vi "StopServer.vi"(8 "error in (no error)":errorcluster, 11 "Server in":refnum<class "Server.lvclass">) -> (0 "error out":errorcluster, 2 "RunTime":u64, 3 "Server out":refnum<class "Server.lvclass">)   [LabVIEW 2017, in "opcua.lvlib" / "Server.lvclass"]
uses:
  Server.lvclass
  Server.lvclass/Server.ctl
  opcua32.dll
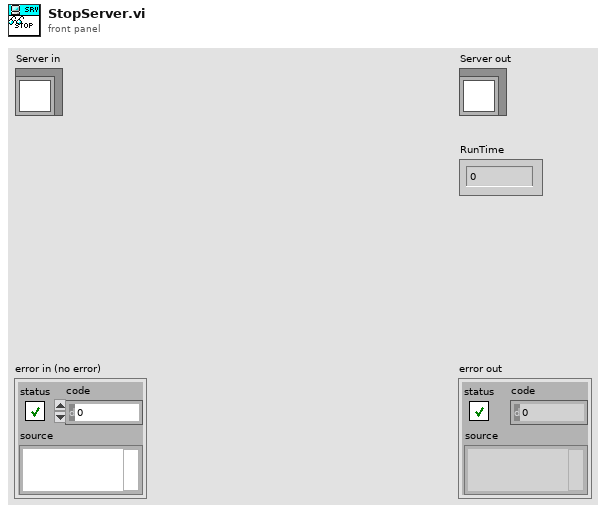
[diagram p1: front panel]
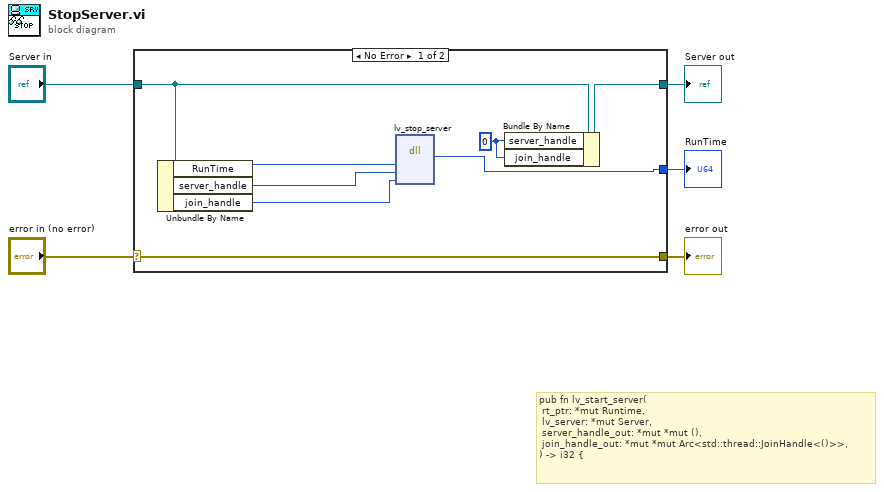
[diagram p0: block diagram]
diagram:
  # "pub fn lv_start_server(\n\trt_ptr: *mut Runtime,\n\tlv_server: *mut Server,\n\tserver_handle_out: *mut *mut (),\n\tjoin_handle_out: *mut *mut Arc<std::thread::JoinHandle<()>>,\n) -> i32 {"
  n1 = case shown="No Error" "error in (no error)" {
    selector: "error in (no error)" -> [w13 w14]
    tunnel: [w13 w14] -> w4
    tunnel: [w9 w15] -> w2
    tunnel: "Server in" -> [w10 w15]
    tunnel: [w8 _] -> w1
    frame No Error {
      w6 = u64 0 ("server_handle")
      n2 = Unbundle By Name(w10) -> ("RunTime"=w12:u64, "server_handle"=w11:u64, "join_handle"=w7:u64)
      n3 = dll-call lib="C:/Users/Andrey/Desktop/opcua-labview/opcua-lvlib/opcua*.dll" fn="lv_stop_server"("RunTime"=w12, "handle"=w11, "joi_handle"=w7) -> ("return type"=w8:i32)  [unwired: 6 in, 2 out]
      n4 = Bundle By Name(cluster=w10, "server_handle"=w6, "join_handle"=w6) -> (w9:refnum<class "Server.lvclass">)
    }
    frame Error {
    }
  }
  "error out" <- w4
  "Server out" <- w2
  "RunTime" <- w1
